vi "ROS_GetPublisherPort.vi"(3 "ROS in":T2) -> (0 "Response":string="<?xml version='1.0'?>\n<methodResponse>\n<params>\n<param>\n<value><array><data>\n<value><int>1</int></value>\n<value><string>Registered [/labview] as publisher of [/robot/head/command_head_nod]</string></value>\n<value><array><data>\n<value><string>http://tuftsBaxter.local:56995/</string></value>\n</data></array></value>\n</data></array></value>\n</param>\n</params>\n</methodResponse>\n", 1 "ROS out":T2)   [LabVIEW 2013]
uses:
  SubVIs/_ROSControl.ctl
  SubVIs/_ROSDirection.ctl
panel:
  in  "Tab Control":enum32{"Text", "Register", "Unregister"}(tab)
  out "unReply":T1
  out "Topic Request":string="POST /RPC2 HTTP/1.1\r\nHost: 192.168.0.101:11311\r\nContent-Type: text/xml\r\nContent-Length: 399\r\n\r\n<?xml version='1.0'?>\n<methodCall>\r <methodName>registerPublisher</methodName>\r <params>\r   <param><value><string>/labview</string> </value> </param>\r   <param><value><string>/robot/head/command_head_nod</string> </value> </param>\r   <param><value><string>std_msgs/Bool</string> </value> </param>\r   <param><value><string>http://192.168.0.102:5000</string> </value> </param>\r </params>\r</methodCall>"
  # "If you register without the listener ready - you will close the port for futher use on Baxter's side"
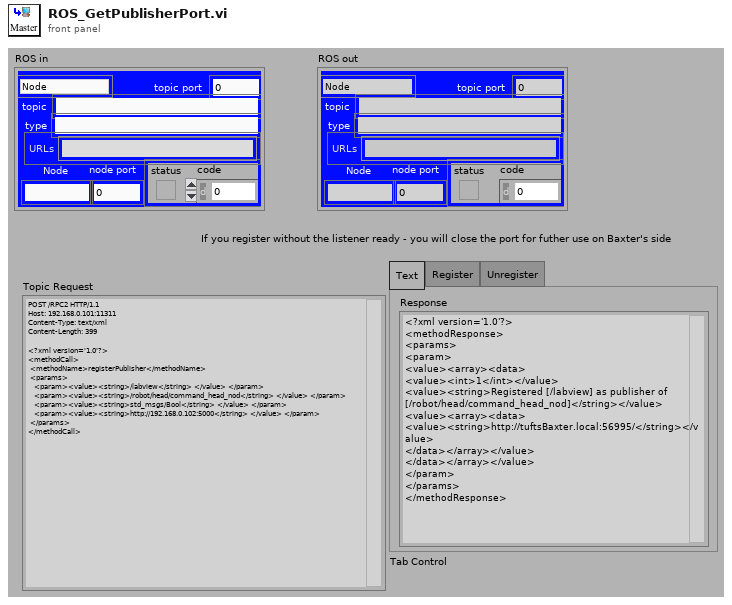
[diagram p1: front panel]
types:
  T1 = cluster{"Code":i8, "statusMessage":string, "APIs":string[]}
  T2 = typedef "_ROSControl.ctl" = cluster{"topic port":u16, "Node":string, "topic":string, "type":string, "node port":u32, "error ":errorcluster, "Direction":T3, "APIs":string[]}
  T3 = typedef "_ROSDirection.ctl" = enum16{"Node", "Publisher", "Subscriber", "Service Client"}
  T4 = cluster{"Caller ID":string, "Topic":string, "Caller API":string}
  T5 = enum16{"http://IP:port", "http://IP", "IP:port", "IP only"}
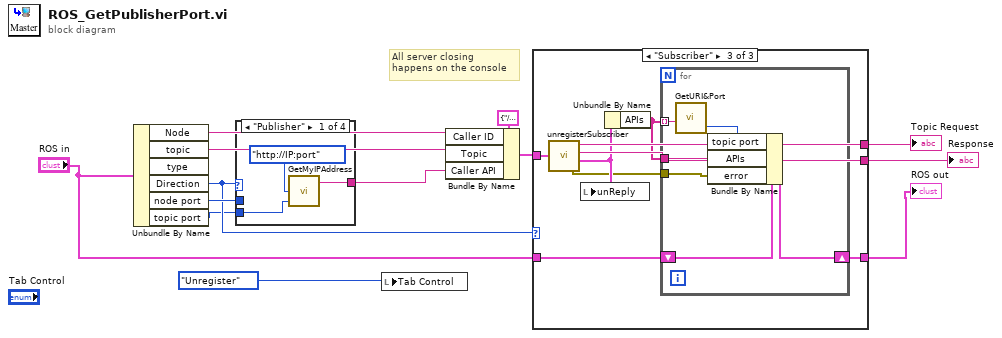
[diagram p0: block diagram]
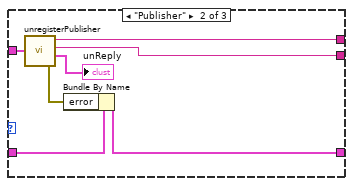
[diagram p3: hidden frame]
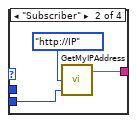
[diagram p4: hidden frame]
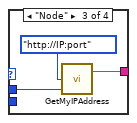
[diagram p5: hidden frame]
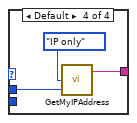
[diagram p6: hidden frame]
diagram:
  # "All server closing\nhappens on the console"
  n1 = Unbundle By Name("ROS in") -> ("Node"=w11:string, "topic"=w10:string, "Direction"=w9:T3, "node port"=w12:u32, "topic port"=w4:u16)  [unwired: 1 out]
  n2 = case shown="\"Publisher\"" w9 {
    tunnel: [w16 w19 w22 w25] -> w8
    tunnel: w12 -> [_ _ w21 w24]
    tunnel: w4 -> [w14 w17 _ _]
    frame "Publisher" {
      n3 = call "GetMyIPAddress.vi"("Port"=w14, "Format"=T5."http://IP:port") -> ("URI"=w16:string)  [unwired: 2 in]
    }
    frame "Subscriber" {
      n4 = call "GetMyIPAddress.vi"("Port"=w17, "Format"=T5."http://IP") -> ("URI"=w19:string)  [unwired: 2 in]
    }
    frame "Node" {
      n5 = call "GetMyIPAddress.vi"("Port"=w21, "Format"=T5."http://IP:port") -> ("URI"=w22:string)  [unwired: 2 in]
    }
    frame Default {
      n6 = call "GetMyIPAddress.vi"("Port"=w24, "Format"=T5."IP only") -> ("URI"=w25:string)  [unwired: 2 in]
    }
  }
  n7 = local write "Tab Control"(enum32{"Text", "Register", "Unregister"}."Unregister" ("Tab Control")) -> ()
  n8 = Bundle By Name(cluster=T4 {"Caller ID"="/labview", "Topic"="/topic", "Caller API"="API"} ("Parameters"), "Caller ID"=w11, "Topic"=w10, "Caller API"=w8) -> (w3:T4)
  n9 = case shown="\"Subscriber\"" w9 {
    tunnel: w3 -> [_ w33 w41]
    tunnel: [_ w32 w40] -> w6
    tunnel: [_ w31 w39] -> w5
    tunnel: "ROS in" -> [w26 w28 w34]
    tunnel: [w26 w27 w38] -> w1
    frame "Node", Default {
    }
    frame "Publisher" {
      n10 = call "unregisterPublisher.vi"("Parameters"=w33) -> ("Error out"=w29:errorcluster, 3:"Reply"=→"unReply":T1, 4:"Reply"=w31:string, "registerPublisher"=w32:string)  [unwired: 1 in]
      n11 = Bundle By Name(cluster=w28, "error"=w29) -> (w27:T2)
    }
    frame "Subscriber" {
      n12 = call "unregisterSubscriber.vi"("Parameters"=w41) -> ("Error out"=w35:errorcluster, 3:"Reply"=w36:T1, 4:"Reply"=w39:string, "registerSubscriber"=w40:string)  [unwired: 1 in]
      n13 = local write "unReply"(w36) -> ()
      n14 = Unbundle By Name(w36) -> ("APIs"=w37:string[])
      n15 = for {
        tunnel: w35 -> [w47]
        tunnel: w37 -> [w46]
        tunnel: w37 -> [w45] mode=indexing
        shift-right: [w42] -> w38
        shift-left: w34 -> [w44]
        n16 = call "GetURI&Port.vi"("URI in"=w45) -> ("Port"=w43:u16)  [unwired: 1 out]
        n17 = Bundle By Name(cluster=w44, "topic port"=w43, "APIs"=w46, "error"=w47) -> (w42:T2)
      }
    }
  }
  "ROS out" <- w1
  "Response" <- w5
  "Topic Request" <- w6
